vi "弹窗-设置.vi"() -> ()   [LabVIEW 2017]
uses:
  cb25fe85-b75d-40f4-990f-57a52c5481f6.vi
panel:
  in  "屏幕键盘":bool
  in  "定时配置":bool
  in  "查看导出":bool
  in  "帮助文档":bool
  in  "远程控制":bool
  in  "退出":bool
  out "信号-关闭窗口":bool=TRUE
  # "定时与导出"
  # "帮助"
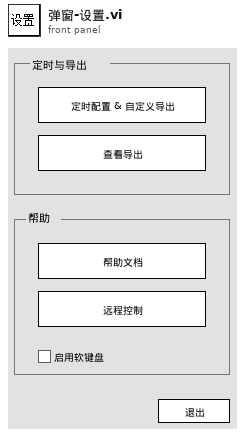
[diagram p1: front panel]
types:
  T1 = typedef "簇-输入.ctl" = cluster{"配置文件动作":T2, "数据输入":variant}
  T2 = typedef "枚举-配置文件动作.ctl" = enum16{"初始化加载配置", "读取配置", "写入-屏幕键盘", "写入-静音延迟", "写入-主要探头类型", "写入-串口配置", "写入-累积定时", "写入-导出定时", "保存配置到文件"}
  T3 = enum32{"Invalid", "Standard", "Closed", "Hidden", "Minimized", "Maximized"}
  T4 = typedef "簇-配置文件内容.ctl" = cluster{"调试模式？":bool, "屏幕键盘？":bool, "软件版本":string, "静音延迟 s":u16, "主要探头类型":T5, "串口配置":cluster{"COM口":refnum<visa-resource-name>, "波特率":enum16{"9600", "19200"}, "读写超时ms":i16, "丢包判定次数":i16}, "定时配置-累积分段":T6, "定时配置-自动导出":cluster{"定时配置-自动导出":T6, "分别导出?":bool}}
  T5 = typedef "枚举-主要探头类型.ctl" = enum16{"网络探头", "串口探头"}
  T6 = typedef "簇-定时配置.ctl" = cluster{"定时模式":enum16{"绝对时间", "相对时间"}, "单位":enum16{"年", "月", "日", "时", "分"}, "间隔":u8, "目标时刻":timestamp}
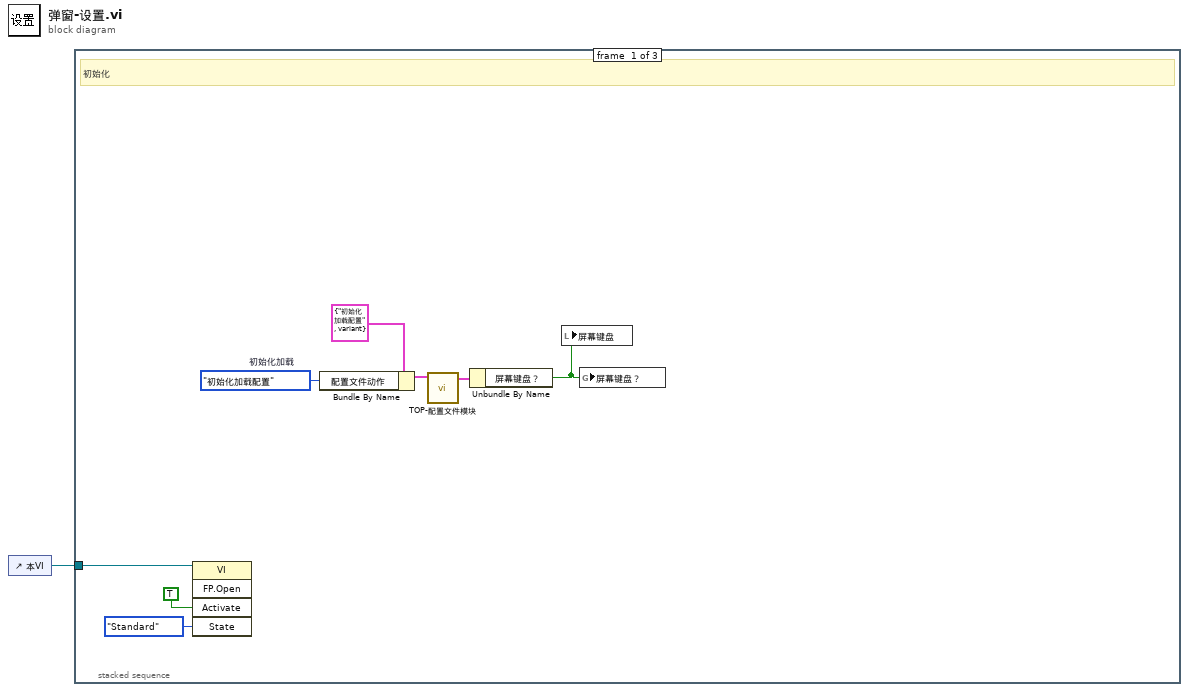
[diagram p0: block diagram]
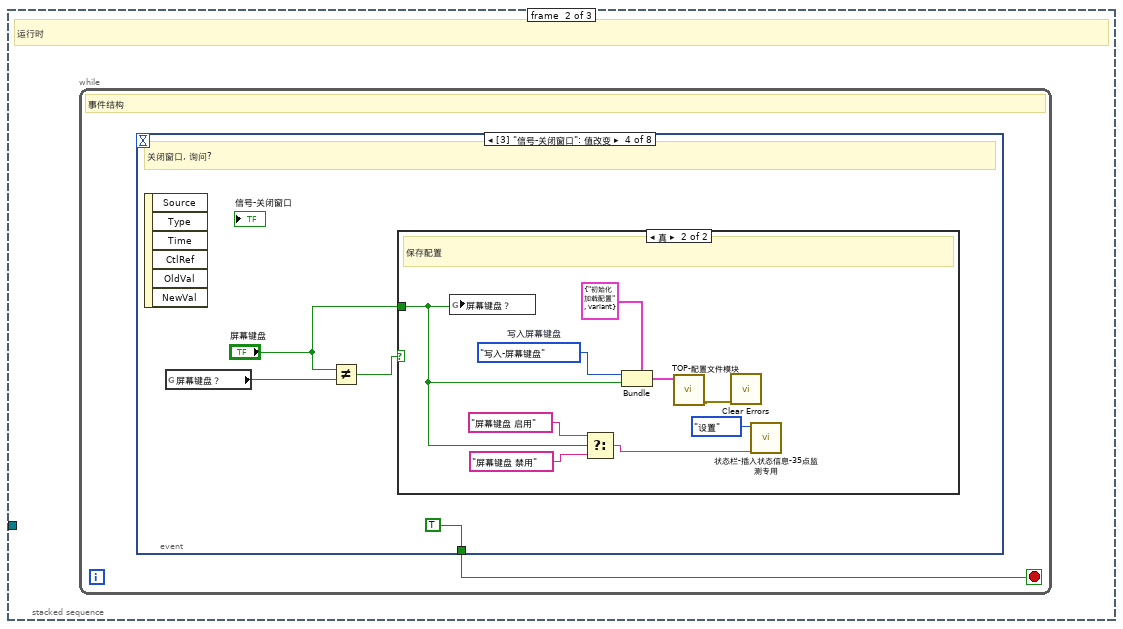
[diagram p2: hidden frame]
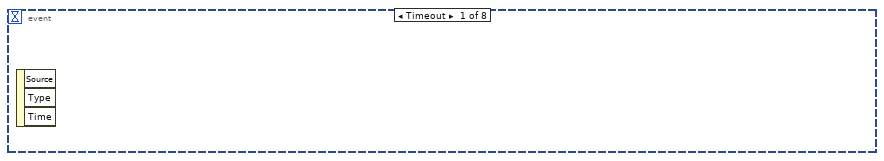
[diagram p3: hidden frame]
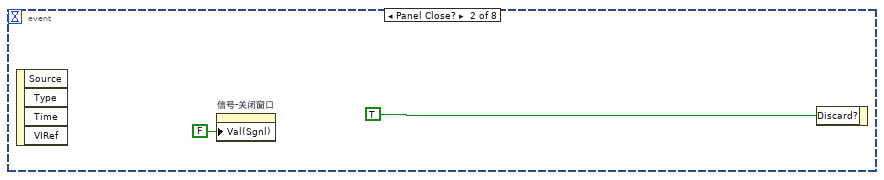
[diagram p4: hidden frame]
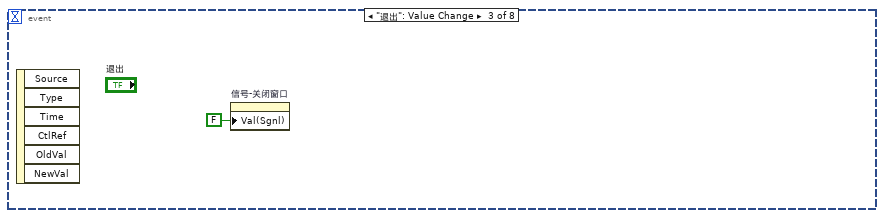
[diagram p5: hidden frame]
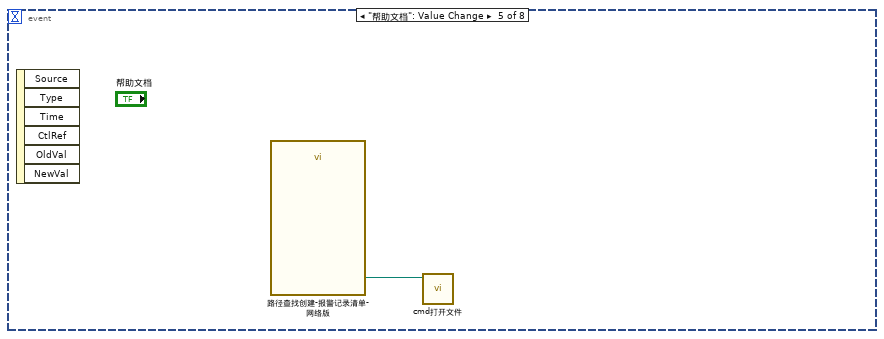
[diagram p7: hidden frame]
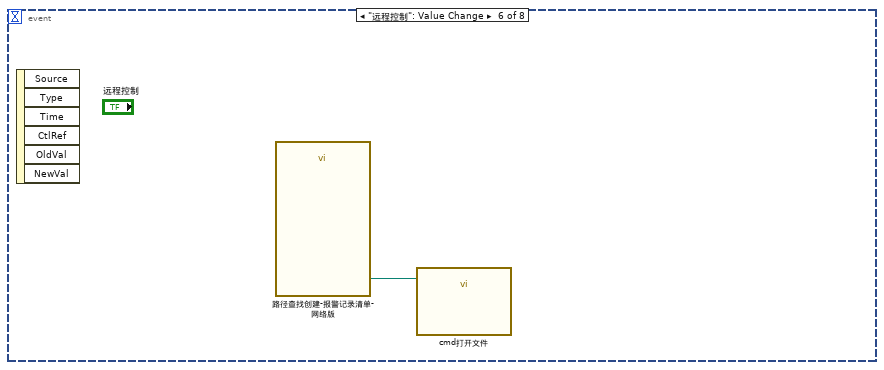
[diagram p8: hidden frame]
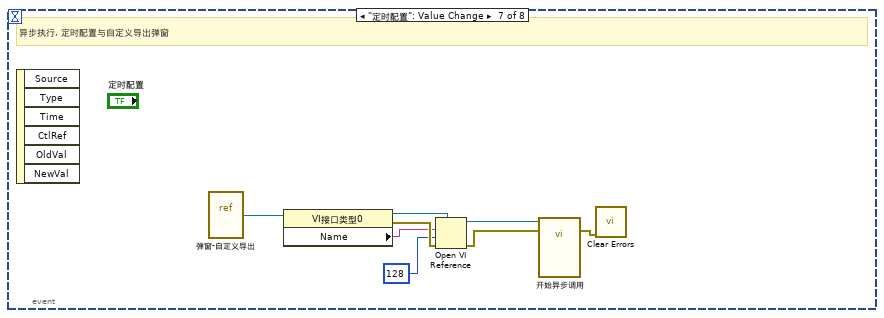
[diagram p9: hidden frame]
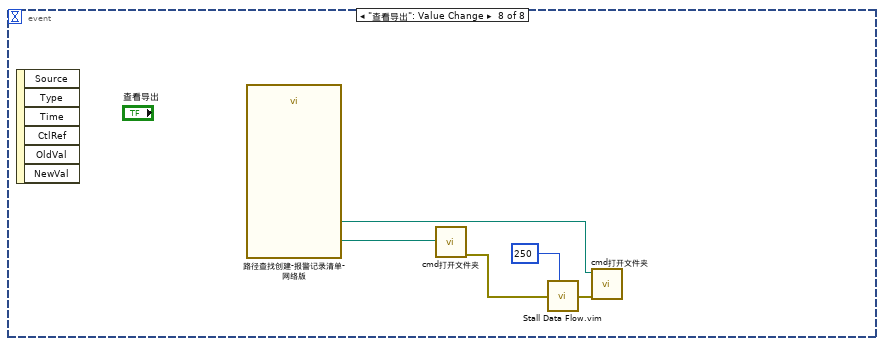
[diagram p10: hidden frame]
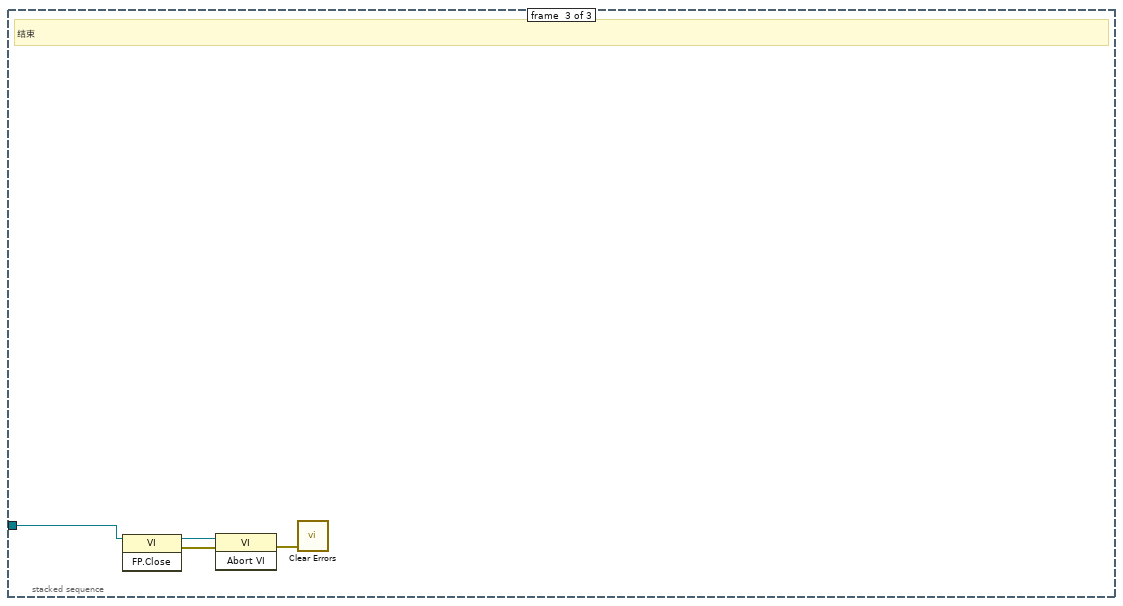
[diagram p11: hidden frame]
diagram:
  n1 = control-ref of="本VI"() -> (w1:refnum<vi>)
  n2 = stacked-sequence {
    tunnel: w1 -> [w9 _ w45]
    frame #0 {
      w4 = 枚举-配置文件动作."初始化加载配置"  # 初始化加载
      # "初始化"
      n3 = invoke class="VI" method="FP.Open"(reference=w9, "Activate"=TRUE ("激活？"), "State"=T3."Standard" ("状态")) -> ()  [unwired: 2 in, 5 out]
      n4 = Bundle By Name(cluster=T1 {"配置文件动作"=enum."初始化加载配置", "数据输入"=variant} ("输入"), "配置文件动作"=w4) -> (w5:T1)
      n5 = call "TOP-配置文件模块.vi"("输入"=w5) -> ("配置文件"=w3:T4)  [unwired: 9 in, 1 out]
      n6 = Unbundle By Name(w3) -> ("屏幕键盘？"=w2:bool)
      n7 = local write "屏幕键盘"(w2) -> ()
      n8 = global write "全局变量-35点监测.vi" "屏幕键盘？"(w2) -> ()
    }
    frame #1 {
      # "运行时"
      n9 = while {
        stop <- w10 stop-if-true
        # "事件结构"
        n10 = event shown="[3] \"信号-关闭窗口\": 值改变" {
          selector: _ -> [_ _ _ _ _ _ _ _]
          dyn-events: _ -> [_ _ _ _ _ _ _ _]
          timeout: _ -> [_ _ _ _ _ _ _ _]
          tunnel: [_ _ _ TRUE _ _ _ _] -> w10
          event Timeout {
            n11 = event-data() -> ()  [unwired: 1 in, 3 out]
          }
          event Panel Close? {
            n12 = event-data() -> ()  [unwired: 1 in, 4 out]
            n13 = property on="信号-关闭窗口" class="Bool (严格)"("Val(Sgnl)"=FALSE ("值(信号)")) -> ()  [unwired: 2 in, 2 out]
            n14 = event-data("Discard?"=TRUE ("放弃？")) -> ()  [unwired: 1 in, 1 out]
          }
          event "退出": Value Change {
            n15 = event-data() -> ()  [unwired: 1 in, 6 out]
            n16 = property on="信号-关闭窗口" class="Bool (严格)"("Val(Sgnl)"=FALSE ("值(信号)")) -> ()  [unwired: 2 in, 2 out]
          }
          event "信号-关闭窗口": Value Change {
            # "关闭窗口, 询问?"
            n17 = event-data() -> ()  [unwired: 1 in, 6 out]
            n18 = global read "全局变量-35点监测.vi" "屏幕键盘？"() -> (w16:bool)
            n19 = Not Equal?(x="屏幕键盘", y=w16) -> (x != y?=w15:bool)
            n20 = case shown="真" w15 {
              tunnel: "屏幕键盘" -> [_ w23]
              frame False {
                # "值未变"
              }
              frame True {
                w25 = 枚举-配置文件动作."写入-屏幕键盘"  # 写入屏幕键盘
                # "保存配置"
                n21 = global write "全局变量-35点监测.vi" "屏幕键盘？"(w23) -> ()
                n22 = Select(t="屏幕键盘 启用" ("消息内容"), s=w23, f="屏幕键盘 禁用" ("消息内容")) -> (s? t:f=w20:string)
                n23 = Bundle(cluster=T1 {"配置文件动作"=enum."初始化加载配置", "数据输入"=variant} ("输入"), "配置文件动作"=w25, "数据输入"=w23) -> (w26:T1)
                n24 = call "TOP-配置文件模块.vi"("输入"=w26) -> ("error out"=w18:errorcluster)  [unwired: 9 in, 1 out]
                n25 = call <vilib>:"Clear Errors.vi"("error in (no error)"=w18) -> ()  [unwired: 5 in, 2 out]
                n26 = call "状态栏-插入状态信息-35点监测专用.vi"("消息内容"=w20, "状态类型"=enum16{"全部", "报警", "通信", "设置"}."设置") -> ()  [unwired: 10 in]
              }
            }
          }
          event "帮助文档": Value Change {
            n27 = event-data() -> ()  [unwired: 1 in, 6 out]
            n28 = call "路径查找创建-报警记录清单-网络版.vi"() -> ("Client 版帮助文档路径"=w27:path)  [unwired: 2 in, 13 out]
            n29 = call "cmd打开文件.vi"("文件路径"=w27) -> ()  [unwired: 10 in, 1 out]
          }
          event "远程控制": Value Change {
            n30 = event-data() -> ()  [unwired: 1 in, 6 out]
            n31 = call "路径查找创建-报警记录清单-网络版.vi"() -> ("远程控制exe"=w28:path)  [unwired: 2 in, 13 out]
            n32 = call "cmd打开文件.vi"("文件路径"=w28) -> ()  [unwired: 10 in, 1 out]
          }
          event "定时配置": Value Change {
            # "异步执行, 定时配置与自定义导出弹窗"
            n33 = event-data() -> ()  [unwired: 1 in, 6 out]
            n34 = vi-ref "弹窗-自定义导出.vi"() -> (w29:refnum<vi>)
            n35 = property class="VI接口类型0"(reference=w29) -> (reference out=w36:refnum<vi>, error out=w33:errorcluster, "Name"=w30:string)  [unwired: 1 in]
            n36 = Open VI Reference(type specifier VI Refnum (for type only)=w36, vi path=w30, options=128 ("选项"), error in (no error)=w33) -> (vi reference=w31:refnum<vi>, error out=w34:errorcluster)  [unwired: 2 in]
            n37 = call-by-ref "开始异步调用"(reference=w31, error in=w34) -> (error out=w35:errorcluster)  [unwired: 12 in, 1 out]
            n38 = call <vilib>:"Clear Errors.vi"("error in (no error)"=w35) -> ()  [unwired: 5 in, 2 out]
          }
          event "查看导出": Value Change {
            n39 = event-data() -> ()  [unwired: 1 in, 6 out]
            n40 = call "路径查找创建-报警记录清单-网络版.vi"() -> ("导出记录"=w37:path, "报表文件夹"=w38:path)  [unwired: 2 in, 12 out]
            n41 = call "cmd打开文件夹.vi"("文件路径"=w38) -> ("error out"=w41:errorcluster)  [unwired: 10 in]
            n42 = call "Stall Data Flow.vim"("value in"=w41, "milliseconds to wait"=u32 250) -> ("value out"=w40:errorcluster)  [unwired: 1 out]
            n43 = call "cmd打开文件夹.vi"("error in (no error)"=w40, "文件路径"=w37) -> ()  [unwired: 9 in, 1 out]
          }
        }
      }
    }
    frame #2 {
      # "结束"
      n44 = invoke class="VI" method="FP.Close"(reference=w45) -> (reference out=w44:refnum<vi>, error out=w43:errorcluster)  [unwired: 2 in, 1 out]
      n45 = invoke class="VI" method="Abort VI"(reference=w44, error in=w43) -> (error out=w42:errorcluster)  [unwired: 1 in, 2 out]
      n46 = call <vilib>:"Clear Errors.vi"("error in (no error)"=w42) -> ()  [unwired: 5 in, 2 out]
    }
  }
